vi "Write Search.vi"(10 "Search":refnum<class "Search.lvclass">, 11 "Dependency in":refnum<class "Dependency.lvclass">) -> (3 "Dependency out":refnum<class "Dependency.lvclass">)   [LabVIEW 2016, in "Dependency.lvclass"]
uses:
  Dependency.lvclass
  Search/Search.lvclass
  Dependency.lvclass/Dependency.ctl
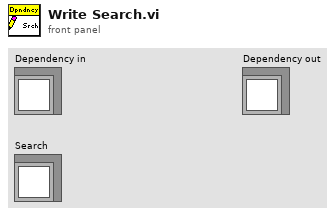
[diagram p1: front panel]
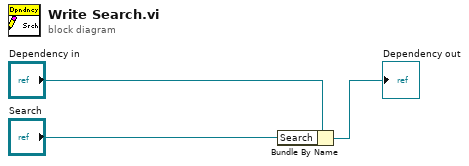
[diagram p0: block diagram]
diagram:
  n1 = Bundle By Name(cluster="Dependency in", "Search"="Search") -> (→"Dependency out":refnum<class "Dependency.lvclass">)
